vi "Limelight enable snapshot.vi"   [LabVIEW 2019]
uses:
  Framework/Robot Global Data.vi
types:
  T1 = typedef "WPI_DriverStationRobotMode2.ctl" = enum16{"Autonomous Disabled", "Autonomous Enabled", "Teleop Disabled", "Teleop Enabled", "Disconnected", "Finish", "Test Disabled", "Test Enabled", "Emergency Stopped"}
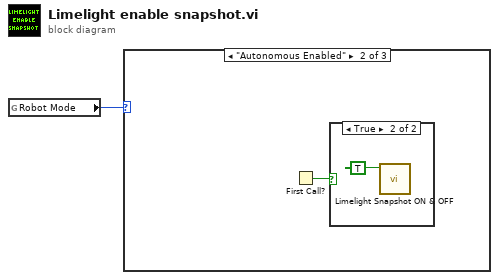
[diagram p0: block diagram]
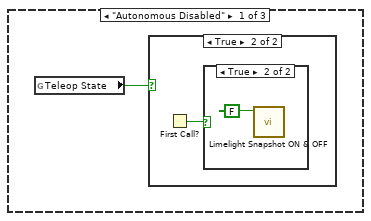
[diagram p2: hidden frame]
diagram:
  n1 = global read "Robot Global Data.vi" "Robot Mode"() -> (w1:T1)
  n2 = case shown="\"Autonomous Enabled\"" w1 {
    frame "Autonomous Disabled" {
      n3 = global read "Robot Global Data.vi" "Teleop State"() -> (w2:bool)
      n4 = case shown="True" w2 {
        frame False {
        }
        frame True {
          n5 = First Call?() -> (First Call?: T/F=w3:bool)
          n6 = case shown="True" w3 {
            frame False {
            }
            frame True {
              n7 = call "Limelight Snapshot ON & OFF.vi"("ON & OFF"=FALSE ("Boolean")) -> ()  [unwired: 10 in, 1 out]
            }
          }
        }
      }
    }
    frame "Autonomous Enabled" {
      n8 = First Call?() -> (First Call?: T/F=w5:bool)
      n9 = case shown="True" w5 {
        frame False {
        }
        frame True {
          n10 = call "Limelight Snapshot ON & OFF.vi"("ON & OFF"=TRUE ("Boolean")) -> ()  [unwired: 10 in, 1 out]
        }
      }
    }
    frame "Teleop Disabled", Default {
    }
  }
